vi "MICSD Reset.vi"(8 "error in (no error)":errorcluster, 11 "VISA Resource Name":refnum<visa-resource-name>) -> (0 "error out":errorcluster, 3 "dup VISA Resource Name":refnum<visa-resource-name>)   [LabVIEW 2020]
uses:
  <vilib>/Instr/_visa.llb/VISA Configure Serial Port (Instr).vi
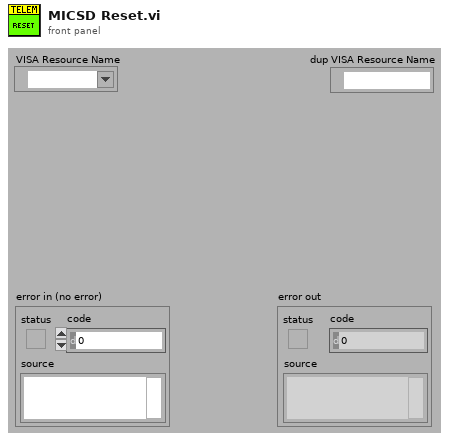
[diagram p1: front panel]
types:
  T1 = cluster{"Command Token":u8, "Length":u16, "Pack Data":u8[]}
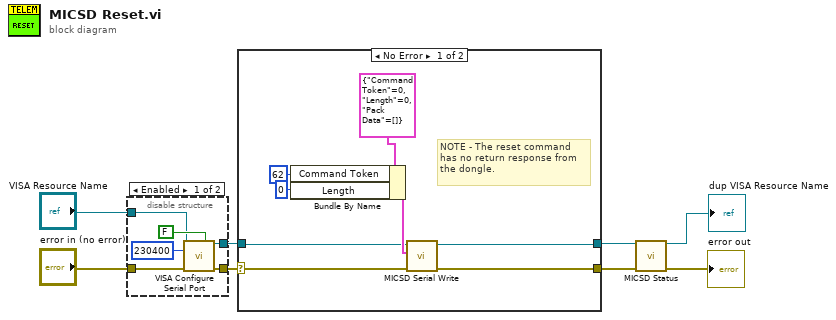
[diagram p0: block diagram]
diagram:
  n1 = disable-structure shown="Enabled" {
    disable-tunnel: [w12 w15] -> w8
    disable-tunnel: [w11 w16] -> w7
    disable-tunnel: "VISA Resource Name" -> [w10 w16]
    disable-tunnel: "error in (no error)" -> [w9 w15]
    frame Enabled {
      n2 = call-poly "VISA Configure Serial Port"("VISA resource name"=w10, "Enable Termination\nChar (T)"=FALSE ("Enable Termination\nChar (T)"), "baud rate (9600)"=u32 230400, "error in (no error)"=w9) -> ("VISA resource name out"=w11:refnum<visa-resource-name>, "error out"=w12:errorcluster)  [unwired: 10 in]
    }
    frame Disabled {
    }
  }
  n3 = case shown="No Error" w8 {
    selector: w8 -> [w20 w26]
    tunnel: [w18 w26] -> w3
    tunnel: w7 -> [w19 w25]
    tunnel: [w17 w25] -> w4
    frame No Error {
      # "NOTE - The reset command\nhas no return response from\nthe dongle."
      n4 = Bundle By Name(cluster=T1 {"Command Token"=0, "Length"=0, "Pack Data"=[]} ("Write Data"), "Command Token"=u8 62, "Length"=u16 0) -> (w24:T1)
      n5 = call "MICSD Serial Write.vi"("error in (no error)"=w20, "Write Data"=w24, "VISA Resource Name"=w19) -> ("error out"=w18:errorcluster, "DUP Visa Resource Name"=w17:refnum<visa-resource-name>)  [unwired: 7 in]
    }
    frame Error {
    }
  }
  n6 = call "MICSD Status.vi"("VISA Resource Name"=w4, "error in (no error)"=w3) -> ("dup VISA Resource Name"=→"dup VISA Resource Name":refnum<visa-resource-name>, "error out"=→"error out":errorcluster)  [unwired: 7 in, 5 out]
